vi "AOTFSettings.vi"(1 "Get/Set":bool, 2 "AOTF Setting (Input)":T1={"Laser 1 Output Channel"="5", "AOTF  1 Output Voltage"=5.0, "Laser 2 Output Channel"="6", "AOTF  2 Output Voltage"=5.0, "Laser 3 Output Channel"="1", "AOTF  3 Output Voltage"=0.0, "Pixel per Cycle"=3, "Time per Cycle  / ms"=0.1, "Laser 4 Output Channel"="1", "AOTF  4 Output Voltage"=0.0} {"AOTF  4 Output Voltage" format="%.2f"; "Time per Cycle  / ms" format="%#.3f"; "AOTF  3 Output Voltage" format="%.2f"; "AOTF  2 Output Voltage" format="%.2f"; "AOTF  1 Output Voltage" format="%.2f"}) -> (0 "AOTF Setting (Output)":T1={"Laser 1 Output Channel"="5", "AOTF  1 Output Voltage"=5.0, "Laser 2 Output Channel"="6", "AOTF  2 Output Voltage"=5.0, "Laser 3 Output Channel"="1", "AOTF  3 Output Voltage"=0.0, "Pixel per Cycle"=3, "Time per Cycle  / ms"=0.1, "Laser 4 Output Channel"="1", "AOTF  4 Output Voltage"=0.0} {"AOTF  4 Output Voltage" format="%.2f"; "Time per Cycle  / ms" format="%#.3f"; "AOTF  3 Output Voltage" format="%.2f"; "AOTF  2 Output Voltage" format="%.2f"; "AOTF  1 Output Voltage" format="%.2f"})   [LabVIEW 2009]
uses:
  AOTFSettings.ctt
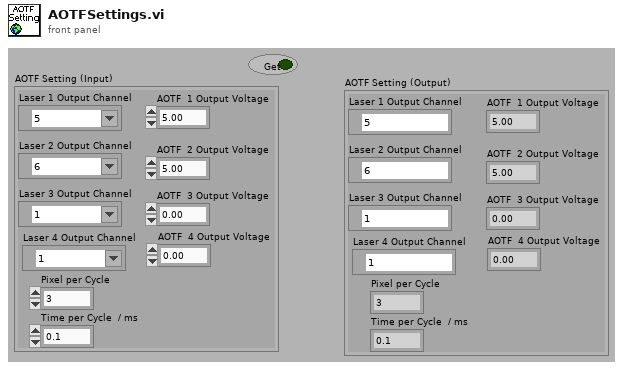
[diagram p1: front panel]
types:
  T1 = typedef "AOTFSettings.ctt" = cluster{"Laser 1 Output Channel":tag, "AOTF  1 Output Voltage":dbl, "Laser 2 Output Channel":tag, "AOTF  2 Output Voltage":dbl, "Laser 3 Output Channel":tag, "AOTF  3 Output Voltage":dbl, "Pixel per Cycle":u16, "Time per Cycle  / ms":dbl, "Laser 4 Output Channel":tag, "AOTF  4 Output Voltage":dbl}
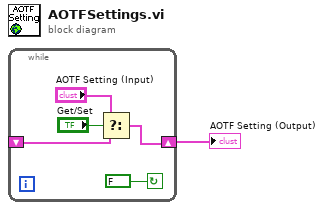
[diagram p0: block diagram]
diagram:
  n1 = while {
    shift-right: [w2] -> w1
    shift-left: _ -> [w5]
    stop <- FALSE continue-if-true
    n2 = Select(t="AOTF Setting (Input)", s="Get/Set", f=w5) -> (s? t:f=w2:T1)
  }
  "AOTF Setting (Output)" <- w1
